vi "Read next.vi"(8 "error in (no error)":errorcluster, 11 "DoublyNode in":refnum<class "DoublyNode.lvclass">) -> (0 "error out":errorcluster, 2 "next":refnum<data-value>, 3 "DoublyNode out":refnum<class "DoublyNode.lvclass">)   [LabVIEW 2021, in "DoublyNode.lvclass"]
uses:
  DoublyNode.lvclass
  IDoublyNode/IDoublyNode.lvclass
  DoublyNode.lvclass/DoublyNode.ctl
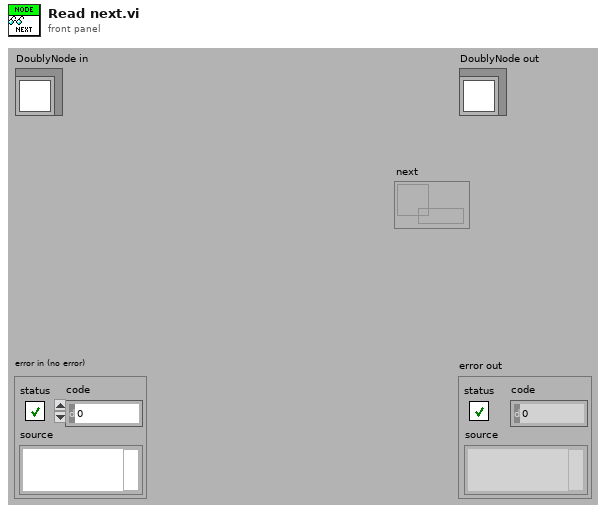
[diagram p1: front panel]
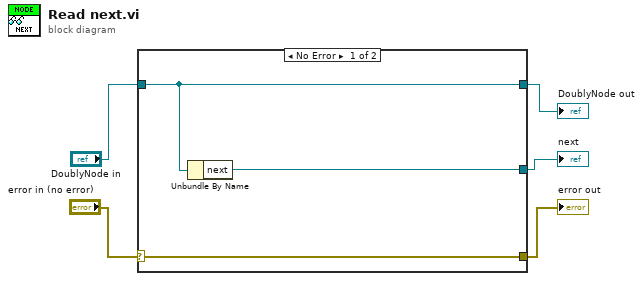
[diagram p0: block diagram]
diagram:
  n1 = case shown="No Error" "error in (no error)" {
    selector: "error in (no error)" -> [w8 w9]
    tunnel: [w8 w9] -> w3
    tunnel: [w7 w10] -> w1
    tunnel: "DoublyNode in" -> [w7 w10]
    tunnel: [w6 _] -> w2
    frame No Error {
      n2 = Unbundle By Name(w7) -> ("next"=w6:refnum<data-value>)
    }
    frame Error {
    }
  }
  "error out" <- w3
  "DoublyNode out" <- w1
  "next" <- w2
